vi "Get Server Connection.vi"(8 "error in (no error)":errorcluster, 11 "TCP Client in":refnum<class "TCP Client.lvclass">) -> (0 "error out":errorcluster, 2 "Server Connection":bool, 3 "TCP Client out":refnum<class "TCP Client.lvclass">)   [LabVIEW 2020, in "Stream-TCP.lvlib" / "TCP Client.lvclass"]
uses:
  TCP Client.lvclass
  TCP Client.lvclass/TCP Client.ctl
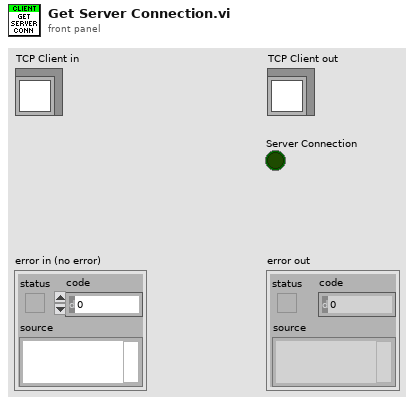
[diagram p1: front panel]
types:
  T1 = typedef "Stream-TCP.lvlib/TCP Client.lvclass/Ref Data.ctl" = cluster{"TCP Connection":refnum<k5>, "TCP Stream":refnum<class "TCP Stream.lvclass">, "State":T2, "Connection Loop":refnum<vi>, "Timeout ms":i32, "Server Connection":bool}
  T2 = typedef "Stream-TCP.lvlib/TCP Client.lvclass/Connection State.ctl" = enum16{"Closed", "Idle", "Connecting", "Connected", "Shutdown"}
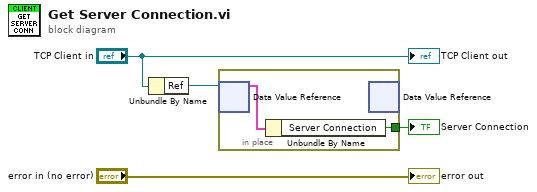
[diagram p0: block diagram]
diagram:
  n1 = Unbundle By Name("TCP Client in") -> ("Ref"=w3:refnum<data-value>)
  n2 = in-place {
    in-place-border: [w5] -> w1
    n3 = in-place-dvr #1(w3) -> (w6:T1)  [unwired: 1 out]
    n4 = Unbundle By Name(w6) -> ("Server Connection"=w5:bool)
    n5 = in-place-dvr #1() -> ()  [unwired: 1 in, 2 out]
  }
  "Server Connection" <- w1
  "error out" <- "error in (no error)"
  "TCP Client out" <- "TCP Client in"
